vi "Generate Error if Invalid.vi"(7 "chain levels to remove (2)":i32=2 min=1, 8 "error in (no error)":errorcluster, 11 "UniCyRO_Host in":refnum<class "UniCyRO_Host.lvclass">) -> (0 "error out":errorcluster, 2 "valid?":bool, 3 "UniCyRO_Host out":refnum<class "UniCyRO_Host.lvclass">)   [LabVIEW 2012, in "UniCyRO.lvlib" / "UniCyRO_Host.lvclass"]
uses:
  UniCyRO_Host.lvclass
  <vilib>/robotics/Utilities/NI_Robotics Utilities.lvlib
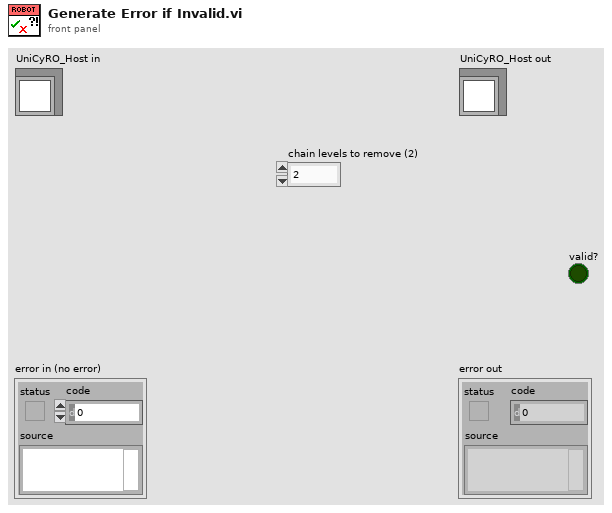
[diagram p1: front panel]
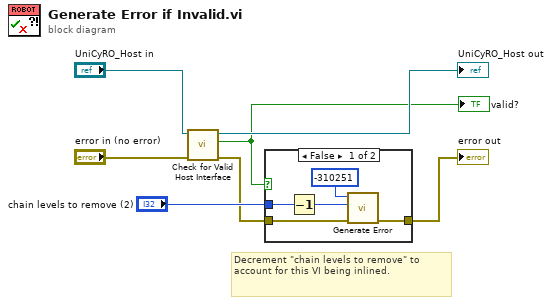
[diagram p0: block diagram]
diagram:
  # "Decrement \"chain levels to remove\" to account for this VI being inlined."
  n1 = call-dynamic "Check for Valid Host Interface.vi"("error in (no error)"="error in (no error)", "UniCyRO_Host in"="UniCyRO_Host in") -> ("error out"=w4:errorcluster, "valid?"=w2:bool, "UniCyRO_Host out"=→"UniCyRO_Host out":refnum<class "UniCyRO_Host.lvclass">)  [unwired: 7 in]
  "valid?" <- w2
  n2 = case shown="False" w2 {
    tunnel: w4 -> [w11 w13]
    tunnel: [w10 w13] -> w1
    tunnel: "chain levels to remove (2)" -> [w9 _]
    frame False {
      n3 = Decrement(x=w9) -> (x-1=w8:i32)
      n4 = call <vilib>:"Generate Error.vi"("error in (no error)"=w11, "chain levels to remove (1)"=w8, "code"=-310251) -> ("error out"=w10:errorcluster)  [unwired: 8 in]
    }
    frame True {
    }
  }
  "error out" <- w1
